vi "RSZVB Check Error.vi"(8 "error in (no error)":errorcluster {"code" format="%.0x"}, 11 "VISA session":refnum<visa-resource-name>) -> (0 "error out":errorcluster {"code" format="%.0x"}, 3 "dup VISA session":refnum<visa-resource-name>)   [LabVIEW 2015]
doc: "This function reads the Standard Event Register and checks it for error. When Error occured, use Error Query VI to describe error type.\n\nRemote-control command(s):\n*ESR?"
uses:
  RSZVB Global Data.vi
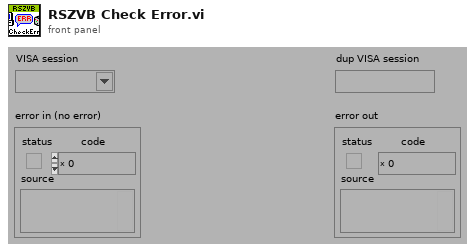
[diagram p1: front panel]
types:
  T1 = cluster{"Error Checking (T: On)":bool, "Installed Options":string[], "Data Valid?":bool, "Ports":i32, "Model":string[], "Option Checking (T: On)":bool}[]
  T2 = cluster{"Error Checking (T: On)":bool, "Installed Options":string[], "Data Valid?":bool, "Ports":i32, "Model":string[], "Option Checking (T: On)":bool}
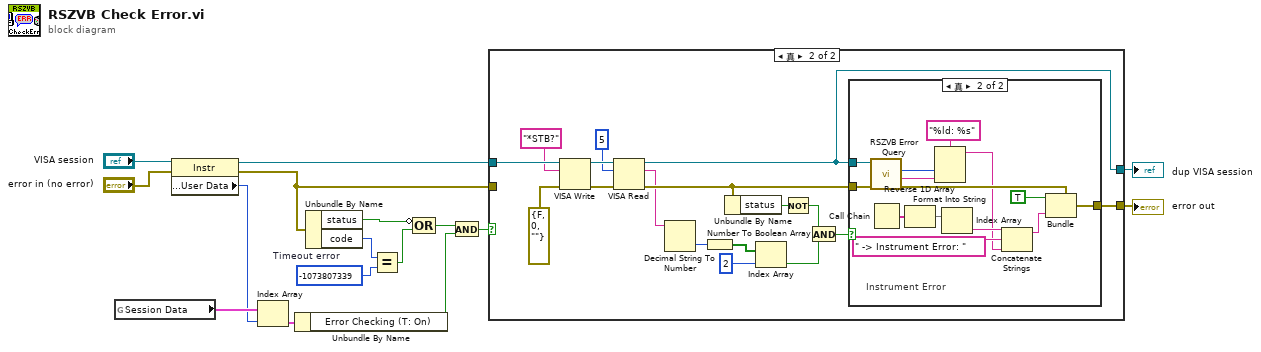
[diagram p0: block diagram]
diagram:
  w6 = -1073807339  # Timeout error
  n1 = global read "RSZVB Global Data.vi" "Session Data"() -> (w11:T1)
  n2 = property class="Instr"(reference="VISA session", error in="error in (no error)") -> (reference out=w12:refnum<visa-resource-name>, error out=w3:errorcluster, "General Settings:User Data"=w10:u32)
  n3 = Index Array(array=w11, index=w10) -> (element=w9:T2)
  n4 = Unbundle By Name(w9) -> ("Error Checking (T: On)"=w2:bool)
  n5 = Unbundle By Name(w3) -> ("status"=w7:bool, "code"=w5:i32)
  n6 = Equal?(x=w5, y=w6) -> (x = y?=w4:bool)
  n7 = Compound Arithmetic op=OR(invert w7, w4) -> (w1:bool)
  n8 = And(x=w1, y=w2) -> (x .and. y?=w8:bool)
  n9 = case shown="真" w8 {
    tunnel: [w17 w33] -> w16
    tunnel: [w18 w27] -> w15
    tunnel: w12 -> [w17 w26]
    tunnel: w3 -> [w18 _]
    frame False {
      # "Communication error or error\nchecking turned off"
    }
    frame True {
      n10 = VISA Write(VISA resource name=w26, write buffer="*STB?" ("write buffer (\"\")"), error in (no error)=errorcluster {"status"=FALSE, "code"=0, "source"=""}) -> (VISA resource name out=w25:refnum<visa-resource-name>, error out=w24:errorcluster)  [unwired: 1 out]
      n11 = VISA Read(VISA resource name=w25, byte count=u32 5 ("byte count (0)"), error in (no error)=w24) -> (VISA resource name out=w33:refnum<visa-resource-name>, read buffer=w21:string, error out=w32:errorcluster)  [unwired: 1 out]
      n12 = Decimal String To Number(string=w21) -> (number=w20:i32)  [unwired: 2 in, 1 out]
      n13 = Number To Boolean Array(number=w20) -> (Boolean array=w35:bool[])
      n14 = Unbundle By Name(w32) -> ("status"=w31:bool)
      n15 = Index Array(array=w35, index=2) -> (element=w28:bool)
      n16 = Not(x=w31) -> (.not. x?=w29:bool)
      n17 = And(x=w29, y=w28) -> (x .and. y?=w30:bool)
      n18 = case shown="真" w30 {
        tunnel: w32 -> [w36 w43]
        tunnel: [w36 w49] -> w27
        tunnel: w33 -> [_ w44]
        frame False {
          # "No Error or IO Error"
        }
        frame True {
          # "Instrument Error"
          n19 = call "RSZVB Error Query.vi"("error in (no error)"=w43, "VISA session"=w44) -> ("error out"=w42:errorcluster, "Error Message"=w38:string, "Error"=w39:i32)  [unwired: 6 in, 1 out]
          n20 = Call Chain() -> (call chain=w48:string[])
          n21 = Reverse 1D Array(array=w48) -> (reversed array=w47:string[])
          n22 = Format Into String(format string="%ld: %s", w39, w38) -> (resulting string=w37:string)  [unwired: 2 in, 1 out]
          n23 = Index Array(array=w47) -> (element=w41:string)  [unwired: 1 in]
          n24 = Concatenate Strings(w41, " -> Instrument Error: " ("string"), w37) -> (w45:string)
          n25 = Bundle(cluster=w42, "status"=TRUE, "source"=w45) -> (w49:errorcluster)  [unwired: 1 in]
        }
      }
    }
  }
  "error out" <- w15
  "dup VISA session" <- w16
